vi "主画面.vi"() -> ()   [LabVIEW 2016]
uses:
  <vilib>/Utility/miscctls.llb/LVPointTypeDef.ctl
  <vilib>/Utility/sysdir.llb/System Directory Type.ctl
  <vilib>/NI/Modbus Library/API/Wrapper/Create TCP Slave.vi
  <vilib>/NI/Modbus Library/API/slave/Modbus Slave.lvclass
  data/FreeMem.dll
  <vilib>/NI/Modbus Library/API/Wrapper/API Main.lvlib
  API/update/update.lvlib
panel:
  in  "关于":bool
  out "SN":string="SN "
  in  "全屏":T1
  out "站点名称":string="站点名称"
  out "时间显示":string="2017-05-09 10:50:42"
  in  "主画面菜单":enum32{"首页", "数据查询", "运维调试", "系统设置"}(xcontrol)
  # "ESTD-XP 地表水水质自动监测系统"
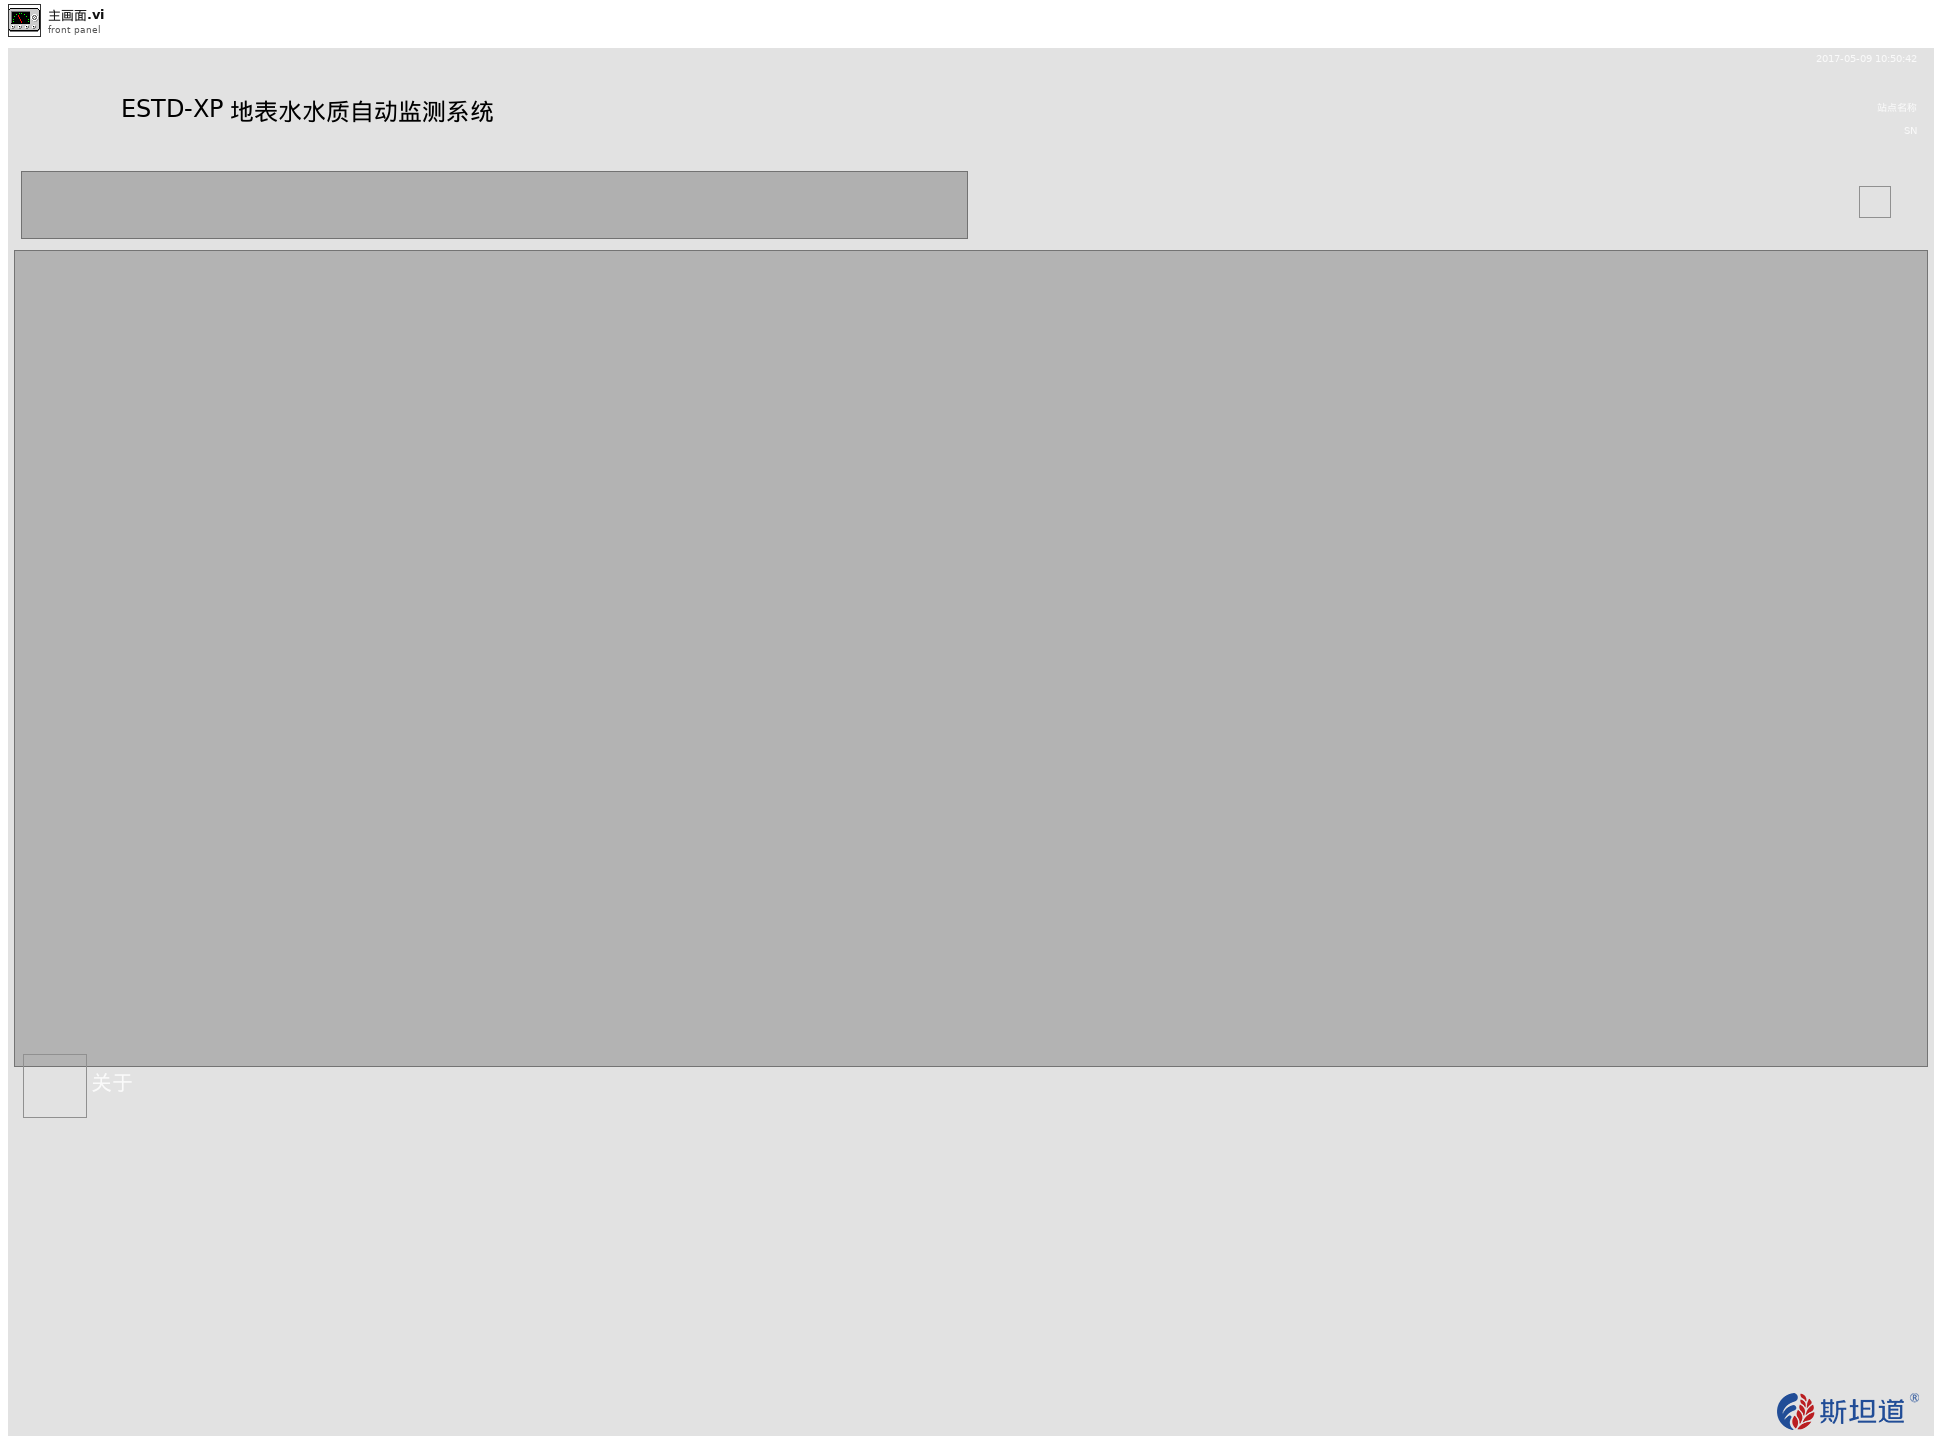
[diagram p1: front panel]
types:
  T1 = typedef "全屏按钮.ctl" = bool
  T2 = typedef "System Directory Type.ctl" = i32
  T3 = typedef "LVPointTypeDef.ctl" = cluster{"Horizontal":i16, "Vertical":i16}
  T4 = cluster{"时间标识":timestamp, "设备":string, "日志信息":string, "流程参数":string}
  T5 = enum32{"Bad", "Idle", "Run top level", "Running"}
  T6 = cluster{"host":string, "user":string, "password":string, "远端地址":string}
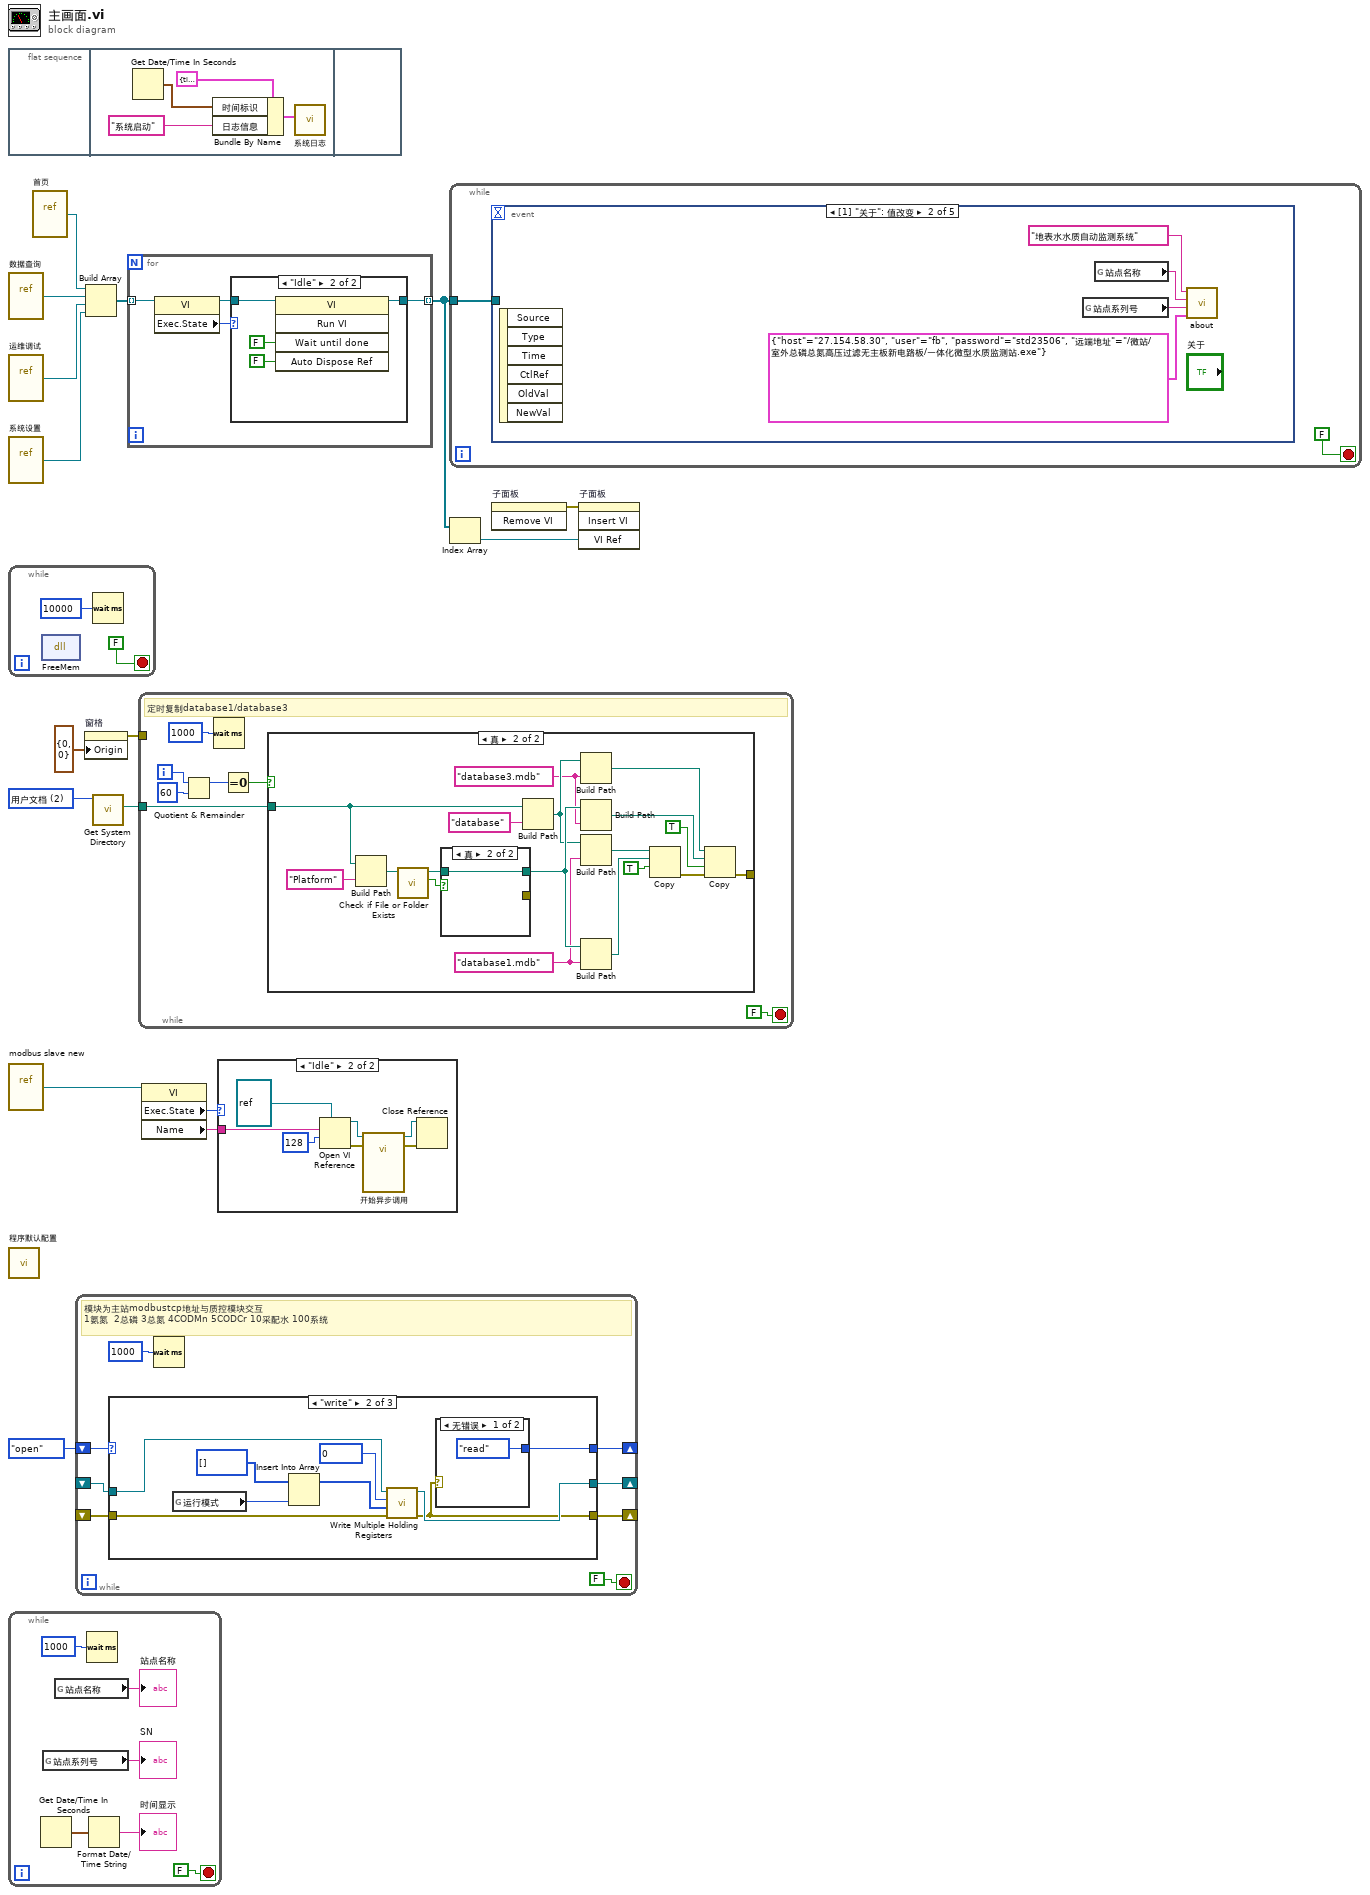
[diagram p0: block diagram]
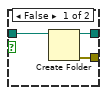
[diagram p3: hidden frame]
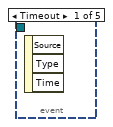
[diagram p6: hidden frame]
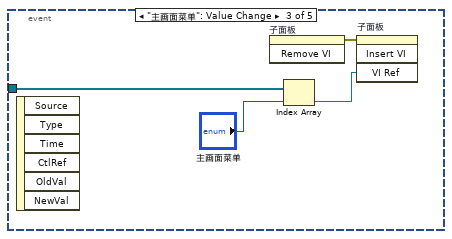
[diagram p7: hidden frame]
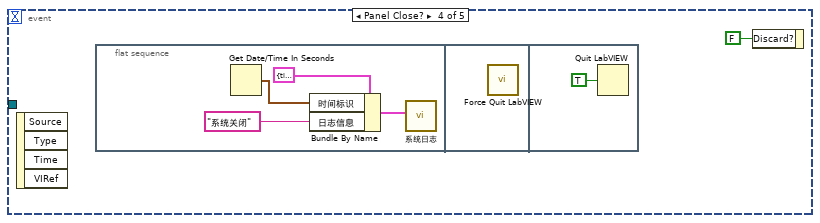
[diagram p8: hidden frame]
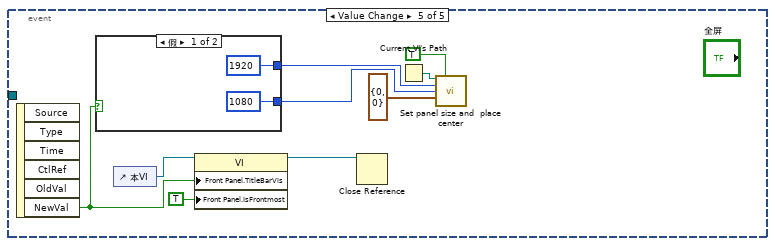
[diagram p9: hidden frame]
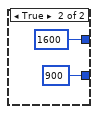
[diagram p10: hidden frame]
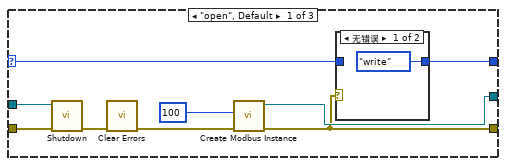
[diagram p11: hidden frame]
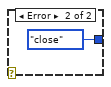
[diagram p13: hidden frame]
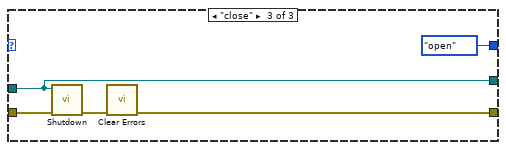
[diagram p14: hidden frame]
diagram:
  w3 = T2 2 items=["用户目录"=0, "用户桌面"=1, "用户文档"=2, "用户应用程序数据"=3, "用户设置"=4, "用户临时目录"=5, "公共文档"=6, "公共应用程序数据"=7, "公共设置"=8, "公共缓存"=13, "系统核心库"=9, "系统安装库"=10, "应用程序文件"=11, "启动盘根目录"=12] ("system directory type")
  n1 = flat-sequence {
    frame #0 {
    }
    frame #1 {
      n2 = Get Date/Time In Seconds() -> (seconds since 1Jan1904=w18:timestamp)
      n3 = Bundle By Name(cluster=T4 {"时间标识"=timestamp(0 s since 1904-01-01), "设备"="系统", "日志信息"="", "流程参数"=""} ("data in"), "时间标识"=w18, "日志信息"="系统启动") -> (w19:T4)
      n4 = call "系统日志.vi"("data in"=w19) -> ()  [unwired: 11 in]
    }
    frame #2 {
    }
  }
  n5 = vi-ref "数据查询.vi"() -> (w10:refnum<vi>)
  n6 = vi-ref "运维调试.vi"() -> (w9:refnum<vi>)
  n7 = vi-ref "系统设置.vi"() -> (w8:refnum<vi>)
  n8 = while {
    stop <- FALSE stop-if-true
    n9 = dll-call lib="PTH2oabs CUsersHsiao\tDocumentsGIT一体站项目模板一体站项目 - 新电路板dataFreeMem.dll" fn="FreeMem"() -> ()  [unwired: 4 in, 2 out]
    n10 = Wait (ms)(milliseconds to wait=u32 10000 ("等待时间（毫秒）")) -> ()  [unwired: 1 out]
  }
  n11 = vi-ref "modbus slave new.vi"() -> (w6:refnum<vi>)
  n12 = call "程序默认配置.vi"() -> ()  [unwired: 11 in, 1 out]
  n13 = while {
    stop <- FALSE stop-if-true
    n14 = Get Date/Time In Seconds() -> (seconds since 1Jan1904=w25:timestamp)
    n15 = global read "系统设置全局变量.vi" "站点系列号"() -> (→"SN":string)
    n16 = global read "系统设置全局变量.vi" "站点名称"() -> (→"站点名称":string)
    n17 = Wait (ms)(milliseconds to wait=u32 1000 ("等待时间（毫秒）")) -> ()  [unwired: 1 out]
    n18 = Format Date/Time String(seconds (now)=w25) -> (date/time string=→"时间显示":string)  [unwired: 2 in]
  }
  n19 = vi-ref "首页.vi"() -> (w11:refnum<vi>)
  n20 = while {
    shift-right: [w34] -> _
    shift-left: _ -> [w36]
    shift-right: [w33] -> _
    shift-left: _ -> [w35]
    shift-right: [w30] -> _
    shift-left: enum16{"open", "read", "write", "close"}."open" -> [w31]
    stop <- FALSE stop-if-true
    # "模块为主站modbustcp地址与质控模块交互\n1氨氮  2总磷 3总氮 4CODMn 5CODCr 10采配水 100系统"
    n21 = case shown="\"write\"" w31 {
      selector: w31 -> [w45 _ _]
      tunnel: w36 -> [w39 w55 w61]
      tunnel: w35 -> [w38 w54 w60]
      tunnel: [w42 w49 w61] -> w34
      tunnel: [w41 w48 w63] -> w33
      tunnel: [w44 w56 enum16{"open", "read", "write", "close"}."open"] -> w30
      frame "open", Default {
        n22 = call-dynamic "Shutdown.vi"("error in"=w38, "Modbus slave in"=w39) -> ("error out"=w37:errorcluster)  [unwired: 9 in]
        n23 = call <vilib>:"Clear Errors.vi"("error in (no error)"=w37) -> ("error out"=w40:errorcluster)  [unwired: 5 in, 1 out]
        n24 = call-poly <vilib>:"Create Modbus Instance.vi"("error in"=w40, "port (502)"=u16 100) -> ("error out"=w41:errorcluster, "TCP slave instance"=w42:refnum<class "Modbus Slave.lvclass">)  [unwired: 8 in]
        n25 = case shown="无错误" w41 {
          tunnel: w45 -> [_ w47]
          tunnel: [enum16{"open", "read", "write", "close"}."write" w47] -> w44
          frame No Error {
          }
          frame Error {
          }
        }
      }
      frame "write" {
        n26 = global read "系统设置全局变量.vi" "运行模式"() -> (w51:enum16{"维护模式", "常规模式", "应急模式", "质控模式"})
        n27 = Insert Into Array(array=u16[] [] ("registers to write"), new element=w51) -> (w50:u16[])  [unwired: 1 in]
        n28 = call-dynamic "Write Multiple Holding Registers.vi"("error in"=w54, "registers to write"=w50, "starting address"=u16 0, "Modbus slave in"=w55) -> ("error out"=w48:errorcluster, "Modbus slave out"=w49:refnum<class "Modbus Slave.lvclass">)  [unwired: 6 in]
        n29 = case shown="无错误" w48 {
          tunnel: [enum16{"open", "read", "write", "close"}."read" enum16{"open", "read", "write", "close"}."close"] -> w56
          frame No Error {
          }
          frame Error {
          }
        }
      }
      frame "close" {
        n30 = call-dynamic "Shutdown.vi"("error in"=w60, "Modbus slave in"=w61) -> ("error out"=w59:errorcluster)  [unwired: 9 in]
        n31 = call <vilib>:"Clear Errors.vi"("error in (no error)"=w59) -> ("error out"=w63:errorcluster)  [unwired: 5 in, 1 out]
      }
    }
    n32 = Wait (ms)(milliseconds to wait=u32 1000 ("等待时间（毫秒）")) -> ()  [unwired: 1 out]
  }
  n33 = property on="窗格" class="Pane"("Origin"=T3 {"Horizontal"=0, "Vertical"=0} ("原点")) -> (error out=w1:errorcluster)  [unwired: 2 in, 1 out]
  n34 = Build Array(w11, w10, w9, w8) -> (w7:refnum<vi>[])
  n35 = call <vilib>:"Get System Directory.vi"("system directory type"=w3) -> ("system directory"=w2:path)  [unwired: 10 in]
  n36 = for {
    tunnel: w7 -> [w67] mode=indexing
    tunnel: [w64] -> w13 mode=indexing
    n37 = property class="VI"(reference=w67) -> (reference out=w65:refnum<vi>, "Exec.State"=w66:T5)  [unwired: 1 in, 1 out]
    n38 = case shown="\"Idle\"" w66 {
      tunnel: w65 -> [w68 w70]
      tunnel: [w68 w69] -> w64
      frame "Bad", Default {
      }
      frame "Idle" {
        n39 = invoke class="VI" method="Run VI"(reference=w70, "Wait until done"=FALSE ("结束前等待"), "Auto Dispose Ref"=FALSE ("自动销毁引用")) -> (reference out=w69:refnum<vi>)  [unwired: 2 in, 4 out]
      }
    }
  }
  n40 = while {
    tunnel: w2 -> [w73]
    tunnel: w1 -> [_]
    i -> [w77]
    stop <- FALSE stop-if-true
    # "定时复制database1/database3"
    n41 = Quotient & Remainder(x=w77, y=60) -> (x-y*floor(x/y)=w75:i32)  [unwired: 1 out]
    n42 = Wait (ms)(milliseconds to wait=u32 1000 ("等待时间（毫秒）")) -> ()  [unwired: 1 out]
    n43 = Equal To 0?(x=w75) -> (x = 0?=w74:bool)
    n44 = case shown="真" w74 {
      tunnel: w73 -> [_ w87]
      tunnel: [_ w83] -> _
      frame False {
      }
      frame True {
        w81 = "database1.mdb" ("名称或相对路径")
        w82 = "database3.mdb" ("名称或相对路径")
        n45 = Build Path(base path=w87, name or relative path="Platform" ("名称或相对路径")) -> (appended path=w94:path)
        n46 = call <vilib>:"Check if File or Folder Exists.vi"("path"=w94) -> ("file or folder exists?"=w93:bool, "dup path"=w92:path)  [unwired: 8 in, 1 out]
        n47 = case shown="真" w93 {
          tunnel: [w99 w101] -> w89
          tunnel: w92 -> [w100 w101]
          tunnel: [w98 _] -> _
          frame False {
            n48 = Create Folder(path (use dialog)=w100) -> (created path=w99:path, error out=w98:errorcluster)  [unwired: 2 in, 1 out]
          }
          frame True {
          }
        }
        n49 = Build Path(base path=w87, name or relative path="database" ("名称或相对路径")) -> (appended path=w85:path)
        n50 = Build Path(base path=w85, name or relative path=w82) -> (appended path=w84:path)
        n51 = Build Path(base path=w89, name or relative path=w82) -> (appended path=w88:path)
        n52 = Build Path(base path=w85, name or relative path=w81) -> (appended path=w86:path)
        n53 = Build Path(base path=w89, name or relative path=w81) -> (appended path=w91:path)
        n54 = Copy(9:TRUE ("覆盖(F)"), 10:w91, 11:w86) -> (0:w90:errorcluster)  [unwired: 2 in, 2 out]
        n55 = Copy(8:w90, 9:TRUE ("覆盖(F)"), 10:w88, 11:w84) -> (0:w83:errorcluster)  [unwired: 1 in, 2 out]
      }
    }
  }
  n56 = property class="VI"(reference=w6) -> ("Exec.State"=w5:T5, "Name"=w4:string)  [unwired: 1 in, 2 out]
  n57 = case shown="\"Idle\"" w5 {
    tunnel: w4 -> [_ w102]
    frame "Bad", Default {
    }
    frame "Idle" {
      n58 = Open VI Reference(type specifier VI Refnum (for type only)=refnum<vi> refnum, vi path=w102, options=128 ("选项")) -> (vi reference=w104:refnum<vi>, error out=w107:errorcluster)  [unwired: 3 in]
      n59 = call-by-ref "开始异步调用"(reference=w104, error in=w107) -> (reference out=w106:refnum<vi>, error out=w108:errorcluster)  [unwired: 12 in]
      n60 = Close Reference(reference=w106, error in (no error)=w108) -> ()  [unwired: 1 out]
    }
  }
  n61 = while {
    tunnel: w13 -> [w109]
    stop <- FALSE stop-if-true
    n62 = event shown="[1] \"关于\": 值改变" {
      selector: _ -> [_ _ _ _ _]
      dyn-events: _ -> [_ _ _ _ _]
      timeout: _ -> [_ _ _ _ _]
      tunnel: w109 -> [_ _ w117 _ _]
      event Timeout {
        n63 = event-data() -> ()  [unwired: 1 in, 3 out]
      }
      event "关于": Value Change {
        n64 = event-data() -> ()  [unwired: 1 in, 6 out]
        n65 = global read "系统设置全局变量.vi" "站点系列号"() -> (w113:string)
        n66 = global read "系统设置全局变量.vi" "站点名称"() -> (w112:string)
        n67 = call "about.vi"("服务器信息"=T6 {"host"="27.154.58.30", "user"="fb", "password"="std23506", "远端地址"="/微站/室外总磷总氮高压过滤无主板新电路板/一体化微型水质监测站.exe"}, "SN输入"=w113, "站点名称输入"=w112, "应用程序名称输入"="地表水水质自动监测系统") -> ()  [unwired: 8 in]
      }
      event "主画面菜单": Value Change {
        n68 = event-data() -> ()  [unwired: 1 in, 6 out]
        n69 = invoke on="子面板" class="SubPnl" method="Remove VI"() -> (error out=w115:errorcluster)  [unwired: 3 in, 2 out]
        n70 = Index Array(array=w117, index="主画面菜单") -> (element=w116:refnum<vi>)
        n71 = invoke on="子面板" class="SubPnl" method="Insert VI"(error in=w115, "VI Ref"=w116) -> ()  [unwired: 2 in, 4 out]
      }
      event Panel Close? {
        n72 = event-data() -> ()  [unwired: 1 in, 4 out]
        n73 = flat-sequence {
          frame #0 {
            n74 = Get Date/Time In Seconds() -> (seconds since 1Jan1904=w122:timestamp)
            n75 = Bundle By Name(cluster=T4 {"时间标识"=timestamp(0 s since 1904-01-01), "设备"="系统", "日志信息"="", "流程参数"=""} ("data in"), "时间标识"=w122, "日志信息"="系统关闭") -> (w121:T4)
            n76 = call "系统日志.vi"("data in"=w121) -> ()  [unwired: 11 in]
          }
          frame #1 {
            n77 = call "Force Quit LabVIEW.vi"() -> ()  [unwired: 10 in, 2 out]
          }
          frame #2 {
            n78 = Quit LabVIEW(quit? (T)=TRUE ("退出？(T)")) -> ()
          }
        }
        n79 = event-data("Discard?"=FALSE ("放弃？")) -> ()  [unwired: 1 in, 1 out]
      }
      event Value Change {
        n80 = event-data() -> ("NewVal"=w128:T1)  [unwired: 1 in, 5 out]
        n81 = case shown="假" w128 {
          tunnel: [1920 ("Panel Width") 1600 ("Panel Width")] -> w127
          tunnel: [1080 ("Panel Height") 900 ("Panel Height")] -> w126
          frame False {
          }
          frame True {
          }
        }
        n82 = control-ref of="本VI"() -> (w133:refnum<vi>)
        n83 = property class="VI"(reference=w133, "Front Panel.TitleBarVis"=w128, "Front Panel.IsFrontmost"=TRUE ("前面板窗口:在最前")) -> (reference out=w129:refnum<vi>)  [unwired: 1 in, 1 out]
        n84 = Close Reference(reference=w129) -> ()  [unwired: 1 in, 1 out]
        n85 = Current VI's Path() -> (path=w132:path)
        n86 = call "Set panel size and  place center.vi"("Path"=w132, "Close Reference (false)"=TRUE, "Panel Width"=w127, "Panel Height"=w126, "FP.Origin in(H & V)"=cluster{"Horizontal":i16, "Vertical":i16} {"Horizontal"=0, "Vertical"=0}) -> ()  [unwired: 6 in, 5 out]
      }
    }
  }
  n87 = Index Array(array=w13) -> (element=w12:refnum<vi>)  [unwired: 1 in]
  n88 = invoke on="子面板" class="SubPnl" method="Remove VI"() -> (error out=w14:errorcluster)  [unwired: 3 in, 2 out]
  n89 = invoke on="子面板" class="SubPnl" method="Insert VI"(error in=w14, "VI Ref"=w12) -> ()  [unwired: 2 in, 4 out]
